vi "YAG_init.v2.vi"(8 "error in (no error)":errorcluster, 9 "initial V":dbl=700.0, 10 "initial rep rate":dbl=10.0, 11 "VISA Refnum in":refnum<visa-resource-name>="COM1") -> (0 "error out":errorcluster={"status"=FALSE, "code"=1073676294, "source"="VISA Read in Cmd-Reply.vi->YAG_init.vi->YAG_Control.v2.vi"}, 3 "VISA Refnum out":refnum<visa-resource-name>="COM1")   [LabVIEW 2018]
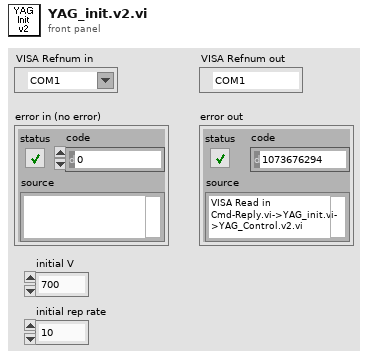
[diagram p1: front panel]
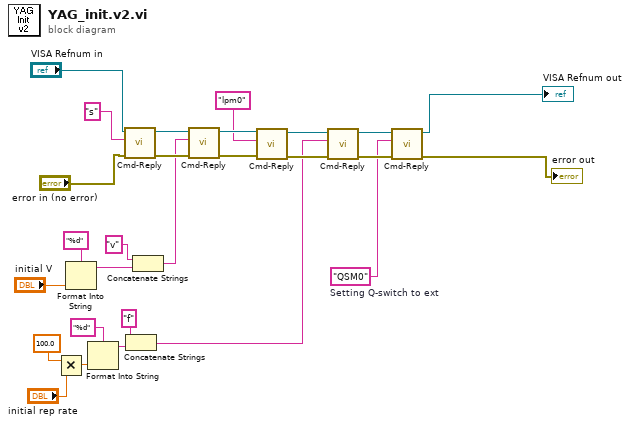
[diagram p0: block diagram]
diagram:
  w1 = "QSM0"  # Setting Q-switch to ext
  n1 = Multiply(x=100.0, y="initial rep rate") -> (x*y=w13:dbl)
  n2 = Format Into String(format string="%d", "initial V") -> (resulting string=w19:string)  [unwired: 2 in, 1 out]
  n3 = Format Into String(format string="%d", w13) -> (resulting string=w11:string)  [unwired: 2 in, 1 out]
  n4 = call "Cmd-Reply.vi"("error in (no error)"="error in (no error)", "cmd"="s", "VISA Refnum in"="VISA Refnum in") -> ("error out"=w24:errorcluster, "VISA Refnum out"=w22:refnum<visa-resource-name>)  [unwired: 6 in, 1 out]
  n5 = Concatenate Strings("f" ("string"), w11) -> (w6:string)
  n6 = Concatenate Strings("v" ("string"), w19) -> (w16:string)
  n7 = call "Cmd-Reply.vi"("error in (no error)"=w24, "cmd"=w16, "VISA Refnum in"=w22) -> ("error out"=w23:errorcluster, "VISA Refnum out"=w21:refnum<visa-resource-name>)  [unwired: 6 in, 1 out]
  n8 = call "Cmd-Reply.vi"("error in (no error)"=w23, "cmd"="lpm0", "VISA Refnum in"=w21) -> ("error out"=w8:errorcluster, "VISA Refnum out"=w9:refnum<visa-resource-name>)  [unwired: 6 in, 1 out]
  n9 = call "Cmd-Reply.vi"("error in (no error)"=w8, "cmd"=w6, "VISA Refnum in"=w9) -> ("error out"=w3:errorcluster, "VISA Refnum out"=w5:refnum<visa-resource-name>)  [unwired: 6 in, 1 out]
  n10 = call "Cmd-Reply.vi"("error in (no error)"=w3, "cmd"=w1, "VISA Refnum in"=w5) -> ("error out"=→"error out":errorcluster, "VISA Refnum out"=→"VISA Refnum out":refnum<visa-resource-name>)  [unwired: 6 in, 1 out]
